vi "Read Tare.vi"(7 "Channel (0: Channel A)":u16(ring) items=["Channel A", "Channel B"], 8 "error in (no error)":errorcluster, 11 "BH Druck PACE Series in":refnum<class "BH Druck PACE Series.lvclass">) -> (0 "error out":errorcluster, 1 "Tare Status":bool, 2 "Tare Value":dbl, 3 "BH Druck PACE Series out":refnum<class "BH Druck PACE Series.lvclass">)   [LabVIEW 2022 SP3, in "BH Druck PACE Series.lvclass"]
uses:
  BH Druck PACE Series.lvclass
  BH Druck PACE Series.lvclass/BH Druck PACE Series.ctl
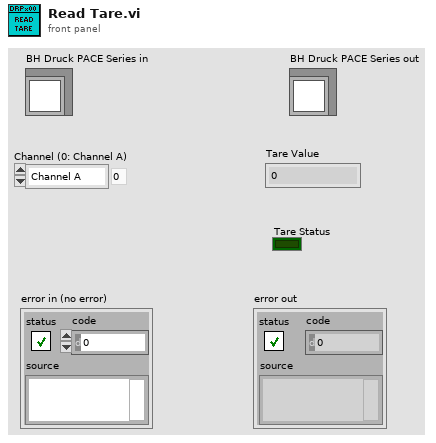
[diagram p1: front panel]
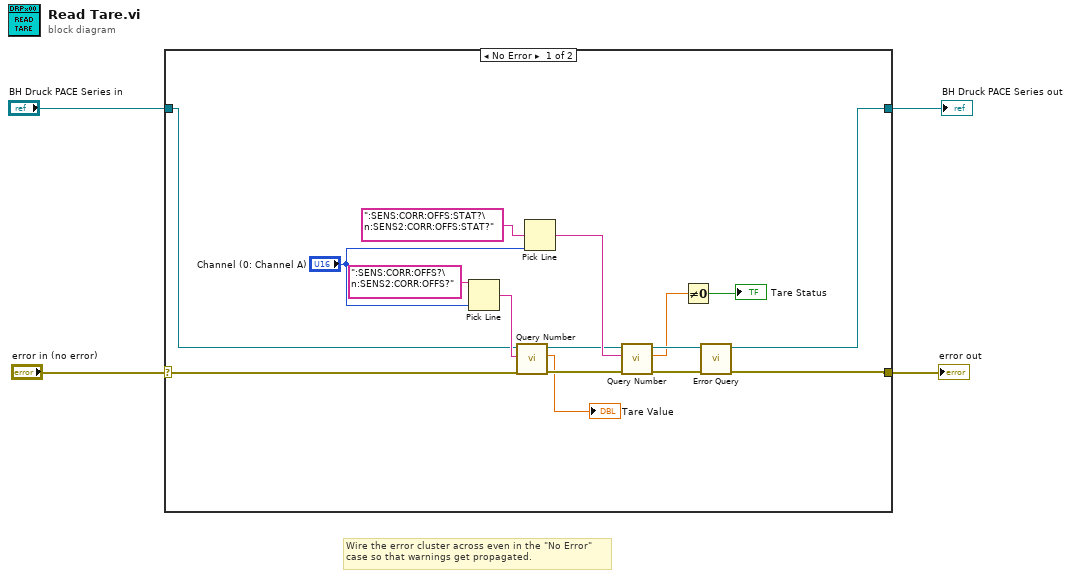
[diagram p0: block diagram]
diagram:
  # "Wire the error cluster across even in the \"No Error\"\ncase so that warnings get propagated."
  n1 = case shown="No Error" "error in (no error)" {
    selector: "error in (no error)" -> [w7 w22]
    tunnel: [w6 w22] -> w3
    tunnel: [w5 w21] -> w1
    tunnel: "BH Druck PACE Series in" -> [w8 w21]
    frame No Error {
      n2 = Pick Line(multi-line string=":SENS:CORR:OFFS?\n:SENS2:CORR:OFFS?", line index="Channel (0: Channel A)") -> (output string=w11:string)  [unwired: 1 in]
      n3 = call-dynamic "Query Number.vi"("error in (no error)"=w7, "Query String"=w11, "BH Druck PACE Series in"=w8) -> ("error out"=w15:errorcluster, "Numeric Result"=→"Tare Value":dbl, "BH Druck PACE Series out"=w14:refnum<class "BH Druck PACE Series.lvclass">)  [unwired: 6 in]
      n4 = Pick Line(multi-line string=":SENS:CORR:OFFS:STAT?\n:SENS2:CORR:OFFS:STAT?", line index="Channel (0: Channel A)") -> (output string=w16:string)  [unwired: 1 in]
      n5 = call-dynamic "Query Number.vi"("error in (no error)"=w15, "Query String"=w16, "BH Druck PACE Series in"=w14) -> ("error out"=w20:errorcluster, "Numeric Result"=w17:dbl, "BH Druck PACE Series out"=w19:refnum<class "BH Druck PACE Series.lvclass">)  [unwired: 6 in]
      n6 = Not Equal To 0?(x=w17) -> (x != 0?=→"Tare Status":bool)
      n7 = call-dynamic "Error Query.vi"("error in (no error)"=w20, "BH Druck PACE Series in"=w19) -> ("error out"=w6:errorcluster, "BH Druck PACE Series out"=w5:refnum<class "BH Druck PACE Series.lvclass">)  [unwired: 8 in]
    }
    frame Error {
    }
  }
  "error out" <- w3
  "BH Druck PACE Series out" <- w1
